vi "Test Ringdown Read.vi"() -> ()   [LabVIEW 2014]
panel:
  out "time stamp":timestamp
  out "Waveform Graph":i16[][](graph)
  out "Array Length":i32[](array[numeric])
  out "offset (in bytes)":i64
  out "Data":i16[](array[numeric])
  out "data":dbl
  out "Numeric Control":i32
  out "error out":errorcluster
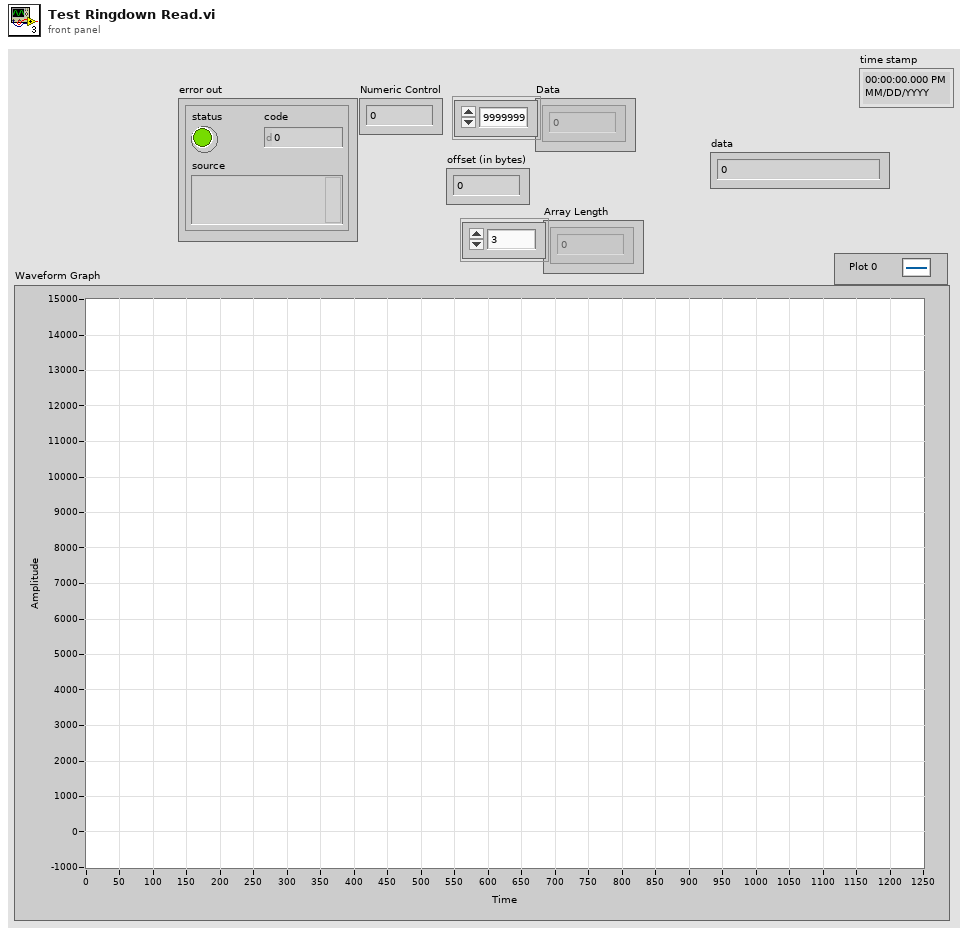
[diagram p1: front panel]
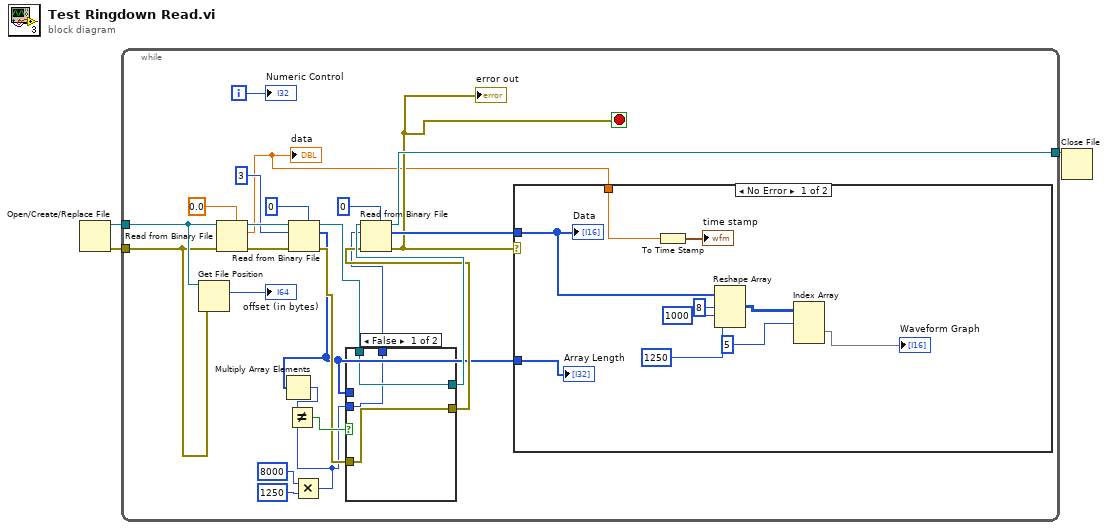
[diagram p0: block diagram]
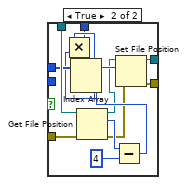
[diagram p2: hidden frame]
diagram:
  n1 = Open/Create/Replace File() -> (refnum out=w3:refnum<file>, error out=w1:errorcluster)  [unwired: 6 in, 1 out]
  n2 = while {
    tunnel: w3 -> [w21]
    tunnel: [w26] -> w2
    tunnel: w1 -> [w20]
    i -> [w27]
    stop <- w14 stop-if-true
    n3 = Get File Position(4:w20, 7:w21) -> (2:→"offset (in bytes)":i64)  [unwired: 2 out]
    n4 = Read from Binary File(5:0.0, 8:w20, 11:w21) -> (0:w17:errorcluster, 2:w13:dbl, 3:w18:refnum<file>)  [unwired: 3 in, 1 out]
    "data" <- w13
    n5 = Read from Binary File(5:0 ("y"), 8:w17, 10:3 ("count (1)"), 11:w18) -> (0:w8:errorcluster, 2:w5:i32[], 3:w10:refnum<file>)  [unwired: 2 in, 1 out]
    n6 = Multiply Array Elements(1:w5) -> (0:w12:i32)
    n7 = Multiply(x=8000, y=1250) -> (x*y=w6:i32)
    n8 = Not Equal?(x=w12, y=w6) -> (x != y?=w11:bool)
    n9 = case shown="False" w11 {
      tunnel: w10 -> [w31 w44]
      tunnel: [w31 w39] -> w9
      tunnel: w8 -> [w30 w38]
      tunnel: [w30 w36] -> w7
      tunnel: w6 -> [w29 _]
      tunnel: w5 -> [_ w35]
      tunnel: [w29 w32] -> w4
      frame False {
      }
      frame True {
        n10 = Index Array(array=w35) -> (element #1=w33:i32, element #2=w34:i32)  [unwired: 2 in]
        n11 = Multiply(x=w33, y=w34) -> (x*y=w32:i32)
        n12 = Get File Position(4:w38, 7:w44) -> (0:w37:errorcluster, 2:w43:i64, 3:w40:refnum<file>)
        n13 = Subtract(x=w43, y=i64 4) -> (x-y=w41:i64)
        n14 = Set File Position(offset (in bytes) (0)=w41, refnum=w40, error in=w37) -> (refnum out=w39:refnum<file>, error out=w36:errorcluster)  [unwired: 1 in]
      }
    }
    n15 = Read from Binary File(5:i16 0, 8:w7, 10:w4, 11:w9) -> (0:w14:errorcluster, 2:w25:i16[], 3:w26:refnum<file>)  [unwired: 2 in, 1 out]
    "error out" <- w14
    n16 = case shown="No Error" w14 {
      tunnel: w25 -> [w54 _]
      tunnel: w13 -> [w46 _]
      tunnel: w5 -> [w45 _]
      frame No Error {
        n17 = To Time Stamp(1:w46) -> (0:→"time stamp":timestamp)
        n18 = Reshape Array(w54, 8 ("dimension size"), 1000 ("dimension size"), 1250 ("dimension size")) -> (w50:i16[][][])
        n19 = Index Array(array=w50, index (dim 0)=5 ("index (page)")) -> (element=→"Waveform Graph":i16[][])  [unwired: 2 in]
        "Data" <- w54
        "Array Length" <- w45
      }
      frame Error {
      }
    }
    "Numeric Control" <- w27
  }
  n20 = Close File(refnum=w2) -> ()  [unwired: 1 in, 2 out]
